vi "test28-MappingRelationshipByExternalRegistration_API_State.vi"(8 "error in (no error)":errorcluster, 11 "TestCase in":refnum<class "testcase-CSMBroadcast.lvclass">) -> (0 "error out":errorcluster, 3 "TestCase out":refnum<class "testcase-CSMBroadcast.lvclass">)   [LabVIEW 2017, in "testcase-CSMBroadcast.lvclass"]
uses:
  testcase-CSMBroadcast.lvclass
  src/user.lib/_NEVSTOP/Communicable State Machine(CSM)/Communicable State Machine.lvlib
  <vilib>/addons/_JKI Toolkits/VI Tester/TestCase.llb/TestCase.lvclass
  CSM/CSM-Testcase.lvlib
  C:/Program Files (x86)/National Instruments/LabVIEW 2017/vi.lib/addons/_JKI Toolkits/VI Tester/TestCase.llb/TestCase.lvclass
panel:
  out "Loop Count":i32
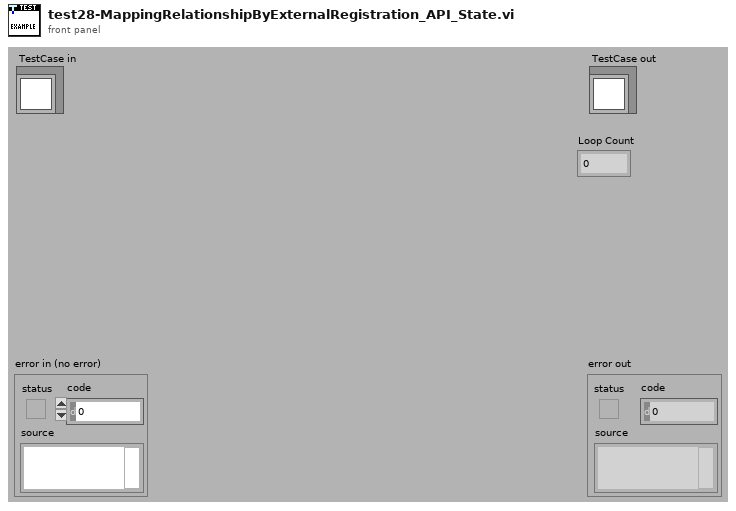
[diagram p1: front panel]
types:
  T1 = cluster{"Status":string, "Source CSM":string, "Target CSM":string, "Target API":string}[]
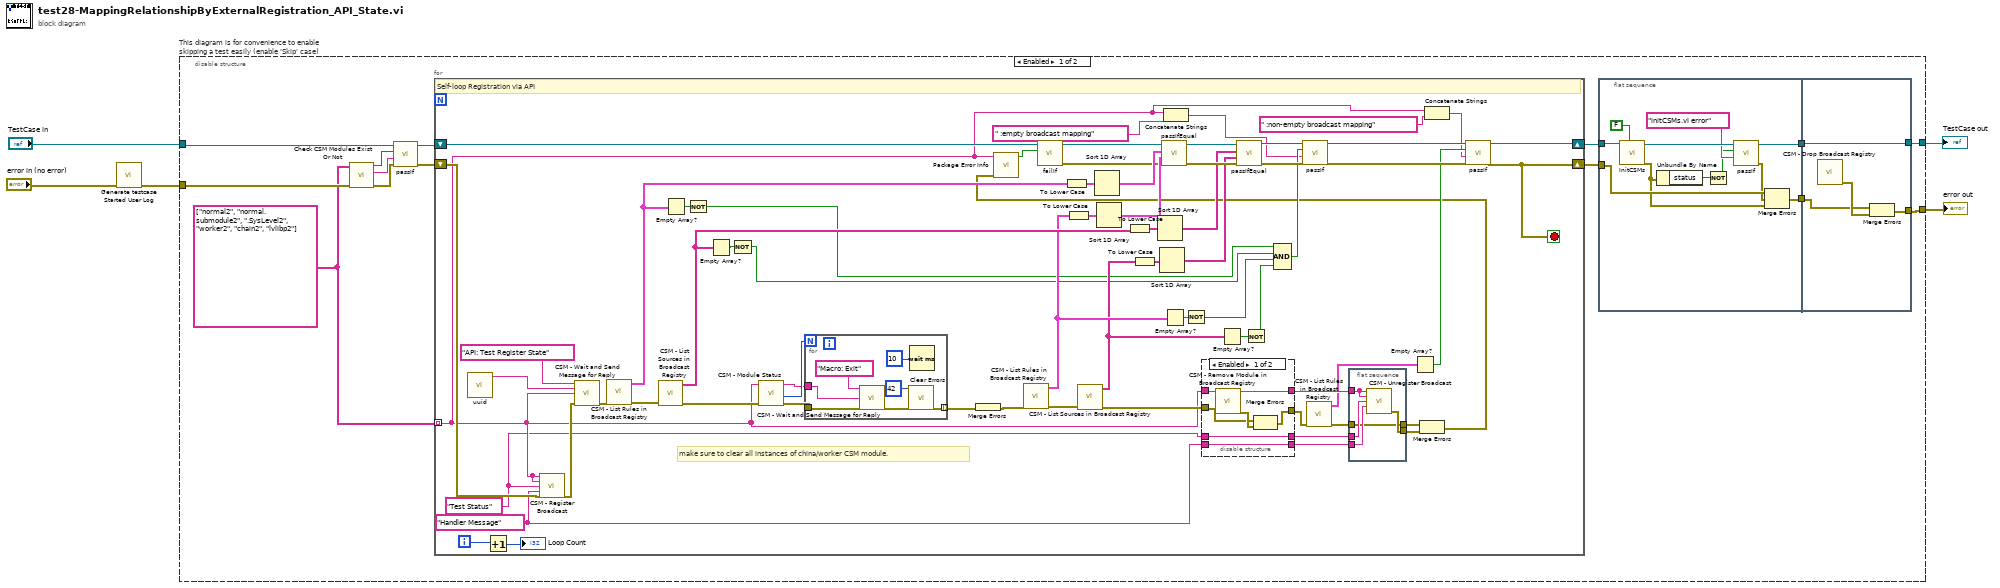
[diagram p0: block diagram]
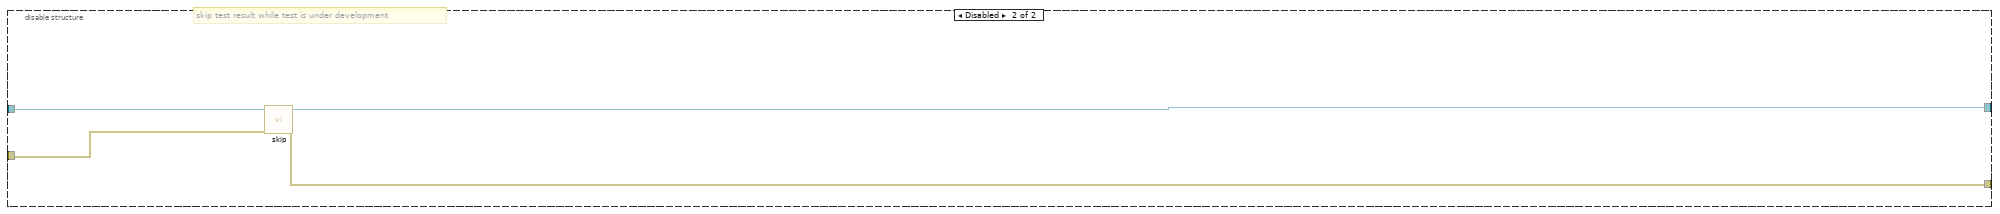
[diagram p3: hidden frame]
diagram:
  n1 = call "Generate testcase Started User Log.vi"("Error In"="error in (no error)") -> ("error out"=w1:errorcluster)  [unwired: 10 in]
  n2 = disable-structure "This diagram is for convenience to enable skipping a test easily (enable 'Skip' case)" shown="Enabled" {
    disable-tunnel: "TestCase in" -> [w16 w127]
    disable-tunnel: [w7 w125] -> w2
    disable-tunnel: [w6 w126] -> w4
    disable-tunnel: w1 -> [w13 w124]
    frame Enabled {
      w12 = string[] ["normal2", "normal.submodule2", ".SysLevel2", "worker2", "chain2", "lvlibp2"]
      n3 = call "Check CSM Modules Exist Or Not.vi"("error in"=w13, "CSM names in"=w12) -> ("error out"=w17:errorcluster, "Debug string"=w18:string, "All Modules Exist?"=w19:bool)  [unwired: 7 in]
      n4 = call-dynamic "passIf.vi"("error in (no error)"=w17, "message (\"\")"=w18, "pass"=w19, "TestCase in"=w16) -> ("error out"=w14:errorcluster, "TestCase out"=w15:refnum<class "testcase-CSMBroadcast.lvclass">)  [unwired: 6 in]
      n5 = for {
        tunnel: w12 -> [w37] mode=indexing
        shift-right: [w64] -> w9
        shift-left: w15 -> [w54]
        shift-right: [w60] -> w8
        shift-left: w14 -> [w61]
        i -> [w83]
        stop <- w60 stop-if-true
        w35 = "Handler Message" ("Response Message (If \"\", Same as Source Message)")
        w36 = "Test Status" ("Status")
        # "make sure to clear all instances of china/worker CSM module."
        # "Self-loop Registration via API"
        n6 = call "uuid.vi"() -> ("UUID"=w99:string)  [unwired: 11 in]
        n7 = Increment(x=w83) -> (x+1=→"Loop Count":i32)
        n8 = call "CSM - Register Broadcast.vi"("CSM Name(Empty for Broadcast Event)"=w37, "Source CSM Name (* as Default)"=w37, "Trigger"=w36, "API (If \"\", Same as Trigger)"=w35, "Error In"=w61) -> ("error out"=w66:errorcluster)  [unwired: 9 in, 1 out]
        n9 = call "CSM - Wait and Send Message for Reply.vi"("State"="API: Test Register State", "Arguments (\"\")"=w99, "Target Module"=w37, "Error In (No Error)"=w66) -> ("error out"=w98:errorcluster)  [unwired: 8 in, 3 out]
        n10 = call "CSM - List Rules in Broadcast Registry.vi"("error in (no error)"=w98) -> ("error out"=w95:errorcluster, "Rule Entries"=w81:T1)  [unwired: 8 in, 1 out]
        n11 = call "CSM - List Sources in Broadcast Registry.vi"("error in (no error)"=w95) -> ("error out"=w56:errorcluster, "Broadcast Names"=w78:string[])  [unwired: 9 in]
        n12 = Empty Array?(array=w81) -> (empty?=w80:bool)
        n13 = Not(x=w80) -> (.not. x?=w73:bool)
        n14 = Empty Array?(array=w78) -> (empty?=w79:bool)
        n15 = Not(x=w79) -> (.not. x?=w72:bool)
        n16 = call "CSM - Module Status.vi"("Error In"=w56, "CSM Name"=w37) -> ("error out"=w57:errorcluster, "#Nodes"=w59:i32, "CSM Name (Dup)"=w58:string)  [unwired: 5 in, 2 out]
        n17 = for {
          N: w59 -> [_]
          tunnel: w58 -> [w121]
          tunnel: w57 -> [w120]
          tunnel: [w119] -> w97 mode=indexing
          n18 = call "CSM - Wait and Send Message for Reply.vi"("State"="Macro: Exit", "Target Module"=w121, "Error In (No Error)"=w120) -> ("error out"=w122:errorcluster)  [unwired: 9 in, 3 out]
          n19 = call <vilib>:"Clear Errors.vi"("error in (no error)"=w122, "specific error code to clear (0: all)"=42) -> ("error out"=w119:errorcluster)  [unwired: 4 in, 1 out]
          n20 = Wait (ms)(milliseconds to wait=u32 10) -> ()  [unwired: 1 out]
        }
        n21 = Merge Errors(w97) -> (w96:errorcluster)
        n22 = call "CSM - List Rules in Broadcast Registry.vi"("error in (no error)"=w96) -> ("error out"=w94:errorcluster, "Rule Entries"=w76:T1)  [unwired: 8 in, 1 out]
        n23 = To Lower Case(string=w81) -> (all lower case string=w93:T1)
        n24 = To Lower Case(string=w76) -> (all lower case string=w92:T1)
        n25 = call "CSM - List Sources in Broadcast Registry.vi"("error in (no error)"=w94) -> ("error out"=w40:errorcluster, "Broadcast Names"=w74:string[])  [unwired: 9 in]
        n26 = Sort 1D Array(array=w93) -> (sorted array=w91:T1)
        n27 = Sort 1D Array(array=w92) -> (sorted array=w90:T1)
        n28 = To Lower Case(string=w78) -> (all lower case string=w87:string[])
        n29 = To Lower Case(string=w74) -> (all lower case string=w86:string[])
        n30 = Sort 1D Array(array=w87) -> (sorted array=w85:string[])
        n31 = Sort 1D Array(array=w86) -> (sorted array=w84:string[])
        n32 = Empty Array?(array=w76) -> (empty?=w77:bool)
        n33 = Concatenate Strings(w37, " :empty broadcast mapping" ("string")) -> (w49:string)
        n34 = Not(x=w77) -> (.not. x?=w71:bool)
        n35 = disable-structure shown="Enabled" {
          disable-tunnel: w40 -> [w106 w115]
          disable-tunnel: [w110 w115] -> w46
          disable-tunnel: w37 -> [w111 w116]
          disable-tunnel: w36 -> [w108 w114]
          disable-tunnel: w35 -> [w107 w113]
          disable-tunnel: [w109 w116] -> w47
          disable-tunnel: [w108 w114] -> w45
          disable-tunnel: [w107 w113] -> w44
          frame Enabled {
            n36 = call "CSM - Remove Module in Broadcast Registry.vi"("CSM Name"=w111) -> ("CSM Name (Dup)"=w109:string, "error out"=w112:errorcluster)  [unwired: 13 in]
            n37 = Merge Errors(w106, w112) -> (w110:errorcluster)
          }
          frame Disabled {
          }
        }
        n38 = Empty Array?(array=w74) -> (empty?=w75:bool)
        n39 = Not(x=w75) -> (.not. x?=w70:bool)
        n40 = Compound Arithmetic op=AND(w73, w72, w71, w70) -> (w67:bool)
        n41 = call "CSM - List Rules in Broadcast Registry.vi"("error in (no error)"=w46) -> ("error out"=w42:errorcluster, "Rule Entries"=w38:T1)  [unwired: 8 in, 1 out]
        n42 = flat-sequence {
          tunnel: w47 -> [w105]
          tunnel: w45 -> [w104]
          tunnel: w44 -> [w103]
          tunnel: [w102] -> w43
          tunnel: w42 -> [w101]
          tunnel: [w101] -> w41
          frame #0 {
            n43 = call "CSM - Unregister Broadcast.vi"("CSM Name(Empty for Broadcast Event)"=w105, "Source CSM Name (* as Default)"=w105, "Trigger"=w104, "API (\"*\" as Default)"=w103) -> ("error out"=w102:errorcluster)  [unwired: 10 in, 1 out]
          }
        }
        n44 = Empty Array?(array=w38) -> (empty?=w62:bool)
        n45 = Merge Errors(w41, w43) -> (w39:errorcluster)
        n46 = call "Package Error Info.vi"("error in"=w39, "String in"=w37) -> ("error status"=w55:bool)  [unwired: 8 in, 1 out]
        n47 = call-dynamic "failIf.vi"("fail"=w55, "TestCase in"=w54) -> ("error out"=w52:errorcluster, "TestCase out"=w53:refnum<class "testcase-CSMBroadcast.lvclass">)  [unwired: 8 in]
        n48 = call-dynamic "passIfEqual.vi"("error in (no error)"=w52, "y"=w90, "x"=w91, "TestCase in"=w53) -> ("error out"=w88:errorcluster, "TestCase out"=w89:refnum<class "testcase-CSMBroadcast.lvclass">)  [unwired: 6 in]
        n49 = call-dynamic "passIfEqual.vi"("error in (no error)"=w88, "y"=w84, "x"=w85, "TestCase in"=w89) -> ("error out"=w68:errorcluster, "TestCase out"=w69:refnum<class "testcase-CSMBroadcast.lvclass">)  [unwired: 6 in]
        n50 = call-dynamic "passIf.vi"("error in (no error)"=w68, "message (\"\")"=w49, "pass"=w67, "TestCase in"=w69) -> ("error out"=w63:errorcluster, "TestCase out"=w65:refnum<class "testcase-CSMBroadcast.lvclass">)  [unwired: 6 in]
        n51 = Concatenate Strings(w37, " :non-empty broadcast mapping" ("string")) -> (w48:string)
        n52 = call-dynamic "passIf.vi"("error in (no error)"=w63, "message (\"\")"=w48, "pass"=w62, "TestCase in"=w65) -> ("error out"=w60:errorcluster, "TestCase out"=w64:refnum<class "testcase-CSMBroadcast.lvclass">)  [unwired: 6 in]
      }
      n53 = flat-sequence {
        tunnel: w9 -> [w30]
        tunnel: [w27] -> w11
        tunnel: w8 -> [w24]
        tunnel: [w21] -> w10
        tunnel: w11 -> [w33]
        tunnel: [w33] -> w7
        tunnel: [w32] -> w6
        tunnel: w10 -> [w31]
        frame #0 {
          n54 = call "InitCSMs.vi"("Enable building lvlibp?"=FALSE, "testcase-CSMStatus in"=w30) -> ("error out"=w22:errorcluster, "testcase-CSMStatus out"=w28:refnum<class "testcase-CSMBroadcast.lvclass">)  [unwired: 8 in]
          n55 = Unbundle By Name(w22) -> ("status"=w26:bool)
          n56 = Not(x=w26) -> (.not. x?=w20:bool)
          n57 = call-dynamic "passIf.vi"("message (\"\")"="initCSMs.vi error" ("message (\"\")"), "pass"=w20, "TestCase in"=w28) -> ("error out"=w23:errorcluster, "TestCase out"=w27:refnum<class "testcase-CSMBroadcast.lvclass">)  [unwired: 7 in]
          n58 = Merge Errors(w24, w23, w22) -> (w21:errorcluster)
        }
        frame #1 {
          n59 = call "CSM - Drop Broadcast Registry.vi"() -> ("error out"=w34:errorcluster)  [unwired: 15 in]
          n60 = Merge Errors(w31, w34) -> (w32:errorcluster)
        }
      }
    }
    frame Disabled {
      # "skip test result while test is under development"
      n61 = call <vilib>:"skip.vi"("error in (no error)"=w124, "TestCase in"=w127) -> ("error out"=w126:errorcluster, "TestCase out"=w125:refnum<class "testcase-CSMBroadcast.lvclass">)  [unwired: 8 in]
    }
  }
  "error out" <- w4
  "TestCase out" <- w2
